vi "FTW-Actor-Initialize.vi"(0 "FTW Actor Instance Type":refnum<class "FTW-ActorInstance.lvclass">, 5 "Initialization Job Sequence":string, 7 "Actor Instance Configuration":string, 11 "error in":errorcluster) -> (4 "FTW Actor Instance":refnum<class "FTW-ActorInstance.lvclass">, 6 "Incoming Requests":refnum<event-registration>, 15 "error out":errorcluster)   [LabVIEW 2013, in "FTW-ActorInstance.lvclass"]
uses:
  FTW-ActorInstance.lvclass
  Message/Request/FTW-Message-IncomingRequest.lvclass
  FTW-Actor-FrameworkEvent.ctl
  FTW-ActorInstance.lvclass/FTW-ActorInstance.ctl
  Endpoint/FTW-Endpoint.lvclass
  Core/src/Reflection/FTW-Reflection-Type.vi
  Core/src/JSON/FTW-JSON-Core-LibraryFilepath.vi
  Core/src/JSON/FTW-JSON-Core-GetFlattenedValue.vi
  Core/src/JSON/FTW-JSON-Core-LibraryError.vi
  Core/utils/CodeGen/JSON Deserialize/FTW-JSON-Deserialize.xnode
  Publisher/FTW-Publisher.lvclass
  JobSequencer/FTW-JobSequencer.lvclass
  Ether/FTW-Ether.lvclass
  Router/FTW-Router.lvclass
panel:
  # "Inputs"
  # "Outputs"
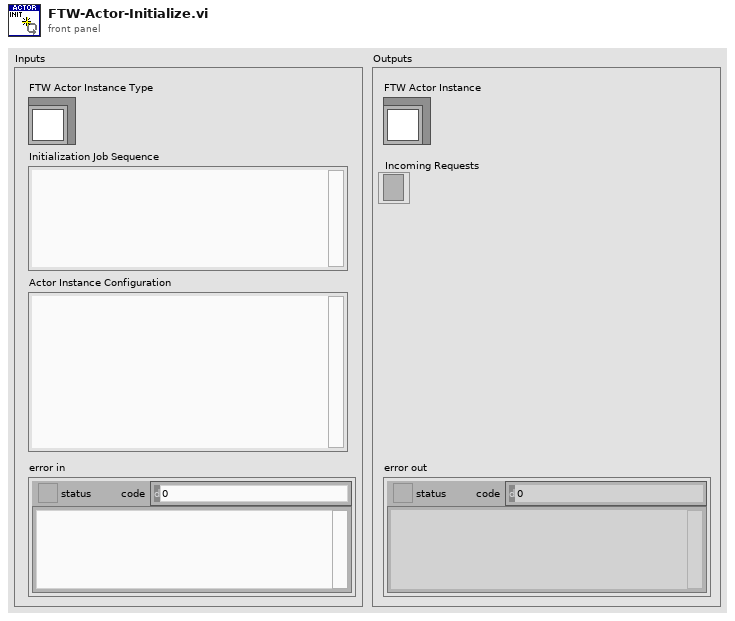
[diagram p1: front panel]
types:
  T1 = typedef "FTW-ActorInstance.lvclass/FTW-Actor-FrameworkEvent.ctl" = enum16{"Instance Initializing", "Instance Initialized", "Instance Job", "Instance Handle Request", "Instance Shutting Down", "Instance Destroyed"}
  T2 = cluster{"Identity":string, "InboxAddress":string, "PublisherAddress":string, "LoggerAddress":string, "DebugEnableInboxLogging":bool, "DebugEnableJobLogging":bool, "LauncherAddress":string}
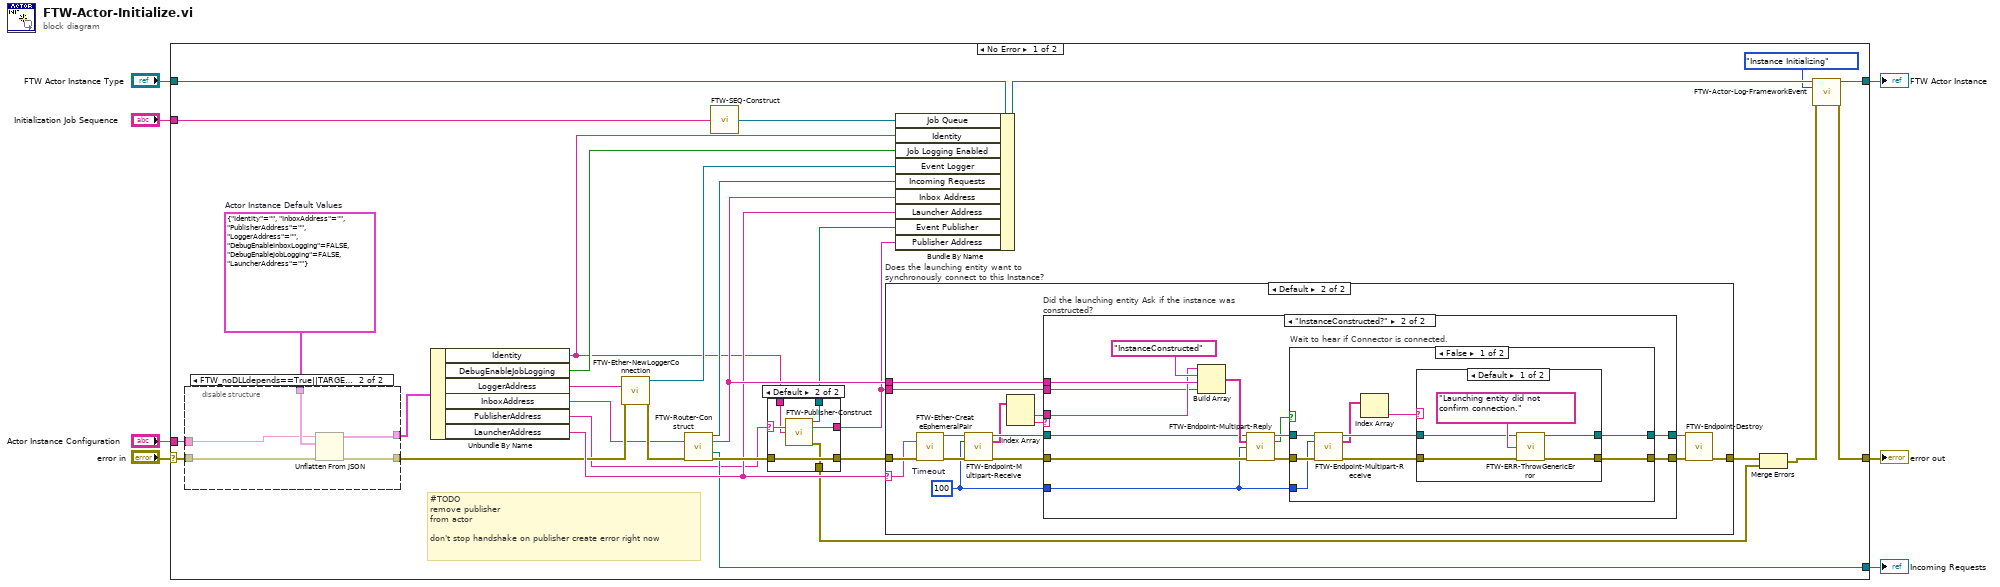
[diagram p0: block diagram]
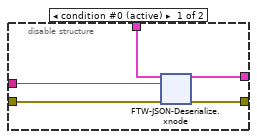
[diagram p2: hidden frame]
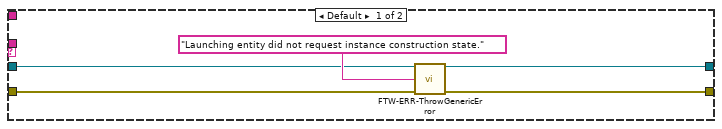
[diagram p5: hidden frame]
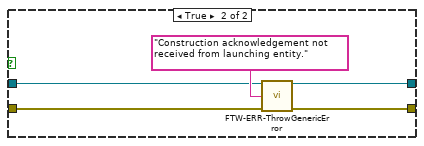
[diagram p7: hidden frame]
diagram:
  n1 = case shown="No Error" "error in" {
    selector: "error in" -> [w24 w142]
    tunnel: "FTW Actor Instance Type" -> [w32 w141]
    tunnel: [w10 w142] -> w6
    tunnel: [w30 _] -> w5
    tunnel: "Initialization Job Sequence" -> [w29 _]
    tunnel: [w15 w141] -> w3
    tunnel: "Actor Instance Configuration" -> [w27 _]
    frame No Error {
      w26 = T2 {"Identity"="", "InboxAddress"="", "PublisherAddress"="", "LoggerAddress"="", "DebugEnableInboxLogging"=FALSE, "DebugEnableJobLogging"=FALSE, "LauncherAddress"=""}  # Actor Instance Default Values
      # "#TODO\nremove publisher\nfrom actor\n\ndon't stop handshake on publisher create error right now"
      n2 = disable-structure shown="FTW_noDLLdepends==True||TARGET_TYPE==RT" {
        disable-tunnel: w27 -> [w42 w78]
        disable-tunnel: w26 -> [w41 w79]
        disable-tunnel: [w40 w77] -> w25
        disable-tunnel: w24 -> [w39 w81]
        disable-tunnel: [w38 w80] -> w23
        frame condition #0 (active) {
          n3 = xnode "FTW-JSON-Deserialize.xnode"("Type and Defaults"=w41, "JSON String"=w42, "error in"=w39) -> ("Values"=w40:T2, "error out"=w38:errorcluster)
        }
        frame condition #1 {
          n4 = Unflatten From JSON(JSON string=w78, type and defaults=w79, error in (no error)=w81) -> (value=w77:T2, error out=w80:errorcluster)  [unwired: 4 in]
        }
      }
      n5 = Unbundle By Name(w25) -> ("Identity"=w8:string, "DebugEnableJobLogging"=w12:bool, "LoggerAddress"=w21:string, "InboxAddress"=w13:string, "PublisherAddress"=w16:string, "LauncherAddress"=w33:string)
      n6 = call "FTW-Ether-NewLoggerConnection.vi"("Logger Address"=w21, "error in"=w23) -> ("Event Logger Connection"=w20:refnum<class "FTW-Logger.lvclass">, "error out"=w22:errorcluster)  [unwired: 12 in]
      n7 = call "FTW-Router-Construct.vi"("Address"=w13, "error in"=w22) -> ("FTW-Router Out"=w35:refnum<class "FTW-Router.lvclass">, "Actual Address"=w37:string, "Event Registration Refnum"=w30:refnum<event-registration>, "error out"=w34:errorcluster)  [unwired: 10 in]
      n8 = call "FTW-SEQ-Construct.vi"("Initial Sequence"=w29) -> ("FTW Job Sequencer"=w36:refnum<class "FTW-JobSequencer.lvclass">)
      n9 = case shown="Default" w16 {
        selector: w16 -> [_ w86]
        tunnel: w34 -> [w82 w85]
        tunnel: [w82 w85] -> w19
        tunnel: [_ w88] -> w18
        tunnel: [_ w87] -> w17
        tunnel: [_ w84] -> w11
        tunnel: w8 -> [_ w83]
        frame "" {
        }
        frame Default {
          n10 = call "FTW-Publisher-Construct.vi"("Address"=w86, "Identity"=w83) -> ("FTW-Publisher Out"=w88:refnum<class "FTW-Publisher.lvclass">, "Actual Address"=w87:string, "error out"=w84:errorcluster)  [unwired: 11 in]
        }
      }
      n11 = case "Does the launching entity want to synchronously connect to this Instance?" shown="Default" w33 {
        selector: w33 -> [_ w91]
        tunnel: w19 -> [w89 w94]
        tunnel: w37 -> [_ w104]
        tunnel: [w89 w97] -> w31
        tunnel: w17 -> [_ w92]
        frame "" {
        }
        frame Default {
          w90 = 100  # Timeout
          n12 = call "FTW-Ether-CreateEphemeralPair.vi"("Requested Ephemeral Address"=w91, "error in"=w94) -> ("Ephemeral Endpoint"=w95:refnum<class "FTW-Endpoint.lvclass">, "error out"=w93:errorcluster)  [unwired: 11 in, 1 out]
          n13 = call-dynamic "FTW-Endpoint-Multipart-Receive.vi"("FTW Endpoint"=w95, "Timeout"=w90, "error in"=w93) -> ("FTW Endpoint out"=w102:refnum<class "FTW-Endpoint.lvclass">, "Message Received"=w101:string[], "error out"=w103:errorcluster)  [unwired: 9 in, 1 out]
          n14 = Index Array(array=w101) -> (element #1=w99:string, element #2=w100:string)  [unwired: 2 in]
          n15 = case "Did the launching entity Ask if the instance was constructed?" shown="\"InstanceConstructed?\"" w100 {
            tunnel: w104 -> [_ w121]
            tunnel: w103 -> [w108 w118]
            tunnel: w102 -> [w105 w117]
            tunnel: w99 -> [_ w116]
            tunnel: [w107 w113] -> w96
            tunnel: [w105 w111] -> w98
            tunnel: w92 -> [_ w110]
            tunnel: w90 -> [_ w109]
            frame Default {
              n16 = call "FTW-ERR-ThrowGenericError.vi"("Error Message"="Launching entity did not request instance construction state.", "error in"=w108) -> ("error out"=w107:errorcluster)  [unwired: 13 in]
            }
            frame "InstanceConstructed?" {
              n17 = Build Array(w116, "InstanceConstructed", w121, w110) -> (w119:string[])
              n18 = call-dynamic "FTW-Endpoint-Multipart-Reply.vi"("FTW Endpoint"=w117, "Multipart Message"=w119, "Timeout"=w109, "error in"=w118) -> ("FTW Endpoint out"=w115:refnum<class "FTW-Endpoint.lvclass">, "Timed out?"=w112:bool, "error out"=w114:errorcluster)  [unwired: 9 in]
              n19 = case "Wait to hear if Connector is connected." shown="False" w112 {
                tunnel: w115 -> [w128 w137]
                tunnel: w114 -> [w126 w139]
                tunnel: w109 -> [w125 _]
                tunnel: [w129 w138] -> w113
                tunnel: [w130 w137] -> w111
                frame False {
                  n20 = call-dynamic "FTW-Endpoint-Multipart-Receive.vi"("FTW Endpoint"=w128, "Timeout"=w125, "error in"=w126) -> ("FTW Endpoint out"=w127:refnum<class "FTW-Endpoint.lvclass">, "Message Received"=w123:string[], "error out"=w124:errorcluster)  [unwired: 9 in, 1 out]
                  n21 = Index Array(array=w123) -> (element=w122:string)  [unwired: 1 in]
                  n22 = case shown="Default" w122 {
                    tunnel: w127 -> [w132 w136]
                    tunnel: w124 -> [w133 w135]
                    tunnel: [w132 w136] -> w130
                    tunnel: [w131 w135] -> w129
                    frame Default {
                      n23 = call "FTW-ERR-ThrowGenericError.vi"("Error Message"="Launching entity did not confirm connection.", "error in"=w133) -> ("error out"=w131:errorcluster)  [unwired: 13 in]
                    }
                    frame "ClientConnected" {
                      # "All is good!"
                    }
                  }
                }
                frame True {
                  n24 = call "FTW-ERR-ThrowGenericError.vi"("Error Message"="Construction acknowledgement not received from launching entity.", "error in"=w139) -> ("error out"=w138:errorcluster)  [unwired: 13 in]
                }
              }
            }
          }
          n25 = call-dynamic "FTW-Endpoint-Destroy.vi"("FTW Endpoint"=w98, "error in"=w96) -> ("error out"=w97:errorcluster)  [unwired: 13 in]
        }
      }
      n26 = Bundle By Name(cluster=w32, "Job Queue"=w36, "Identity"=w8, "Job Logging Enabled"=w12, "Event Logger"=w20, "Incoming Requests"=w35, "Inbox Address"=w37, "Launcher Address"=w33, "Event Publisher"=w18, "Publisher Address"=w17) -> (w28:refnum<class "FTW-ActorInstance.lvclass">)
      n27 = Merge Errors(w31, w11) -> (w9:errorcluster)
      n28 = call "FTW-Actor-Log-FrameworkEvent.vi"("FTW Actor Instance"=w28, "Framework Event"=FTW-Actor-FrameworkEvent."Instance Initializing", "error in"=w9) -> ("FTW Actor Instance out"=w15:refnum<class "FTW-ActorInstance.lvclass">, "error out"=w10:errorcluster)  [unwired: 11 in]
    }
    frame Error {
    }
  }
  "FTW Actor Instance" <- w3
  "error out" <- w6
  "Incoming Requests" <- w5
